vi "Dictionary Set Modified Data__ogtk.vi"(8 "error in (no error)":errorcluster, 10 "Data in":T2, 11 "Object RefNum":T1) -> (0 "error out":errorcluster, 3 "dup Object RefNum":T1)   [LabVIEW 2019]
doc: "Sets the GOOP data structure and releases mutex"
uses:
  Dictionary Object Data Core Task Enum__ogtk.ctl
  Dictionary Data__ogtk.ctl
  Dictionary Object RefNum - Enum__ogtk.ctl
  Dictionary Object RefNum__ogtk.ctl
panel:
  # "OpenGOOP Set Modified Data.vi\n\nSets the GOOP data structure and releases mutex\n\nPlease visit http://www.OpenG.org to learn about the\nOpen Source LabVIEW software movement.\n\nNOTICE -- YOU MUST LEAVE THIS NOTICE IN PLACE.  PER THE TERMS OF THE LICENSE BELOW, YOU MAY SUBLICENSE THIS SOFTWARE \nIN ANY WAY THAT DOES NOT CONFLICT WITH THIS LICENSE.\n\n### BSD License (http://www.opensource.org/licenses/bsd-license.php) Begin ###\n \nCopyright (c) 2003, Jim Kring <jim@jimkring.com>\n\nAll rights reserved.\n\nRedistribution and use in source and binary forms, with or without modification, are permitted provided that the following conditions are met:\n\n    * Redistributions of source code must retain the above copyright notice, this list of conditions and the following disclaimer.\n    * Redistributions in binary form must reproduce the above copyright notice, this list of conditions and the following disclaimer in the \n       documentation and/or other materials provided with the distribution.\n    * Neither the name of SciWare, James Kring, Inc., nor the names of its contributors may be used to endorse or promote products derived \n       from this software without specific prior written permission.\n\nTHIS SOFTWARE IS PROVIDED BY THE COPYRIGHT HOLDERS AND CONTRIBUTORS \"AS IS\" AND ANY EXPRESS OR IMPLIED WARRANTIES, \nINCLUDING, BUT NOT LIMITED TO, THE IMPLIED WARRANTIES OF MERCHANTABILITY AND FITNESS FOR A PARTICULAR PURPOSE ARE \nDISCLAIMED. IN NO EVENT SHALL THE COPYRIGHT OWNER OR CONTRIBUTORS BE LIABLE FOR ANY DIRECT, INDIRECT, INCIDENTAL,\n SPECIAL, EXEMPLARY, OR CONSEQUENTIAL DAMAGES (INCLUDING, BUT NOT LIMITED TO, PROCUREMENT OF SUBSTITUTE GOODS OR \nSERVICES; LOSS OF USE, DATA, OR PROFITS; OR BUSINESS INTERRUPTION) HOWEVER CAUSED AND ON ANY THEORY OF LIABILITY, \nWHETHER IN CONTRACT, STRICT LIABILITY, OR TORT (INCLUDING NEGLIGENCE OR OTHERWISE) ARISING IN ANY WAY OUT OF THE USE \nOF THIS SOFTWARE, EVEN IF ADVISED OF THE POSSIBILITY OF SUCH DAMAGE.\n\n### BSD License End ###"
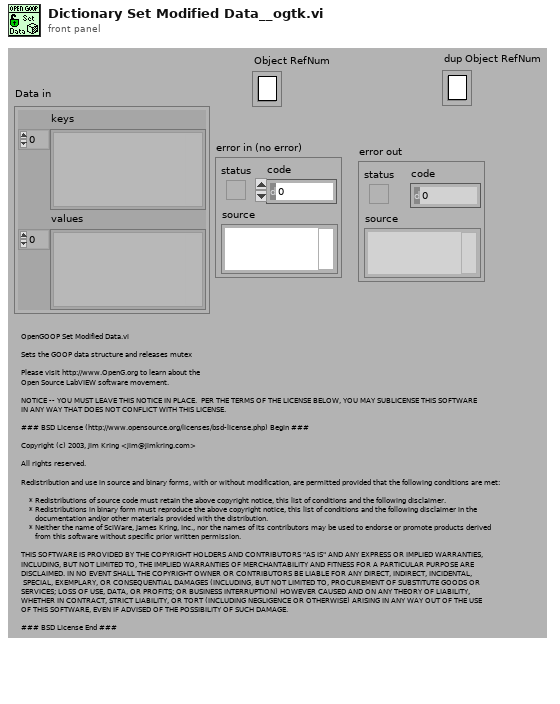
[diagram p1: front panel]
types:
  T1 = typedef "Dictionary Object RefNum__ogtk.ctl" = refnum<k1>
  T2 = typedef "Dictionary Data__ogtk.ctl" = cluster{"keys":variant[], "values":variant[]}
  T3 = typedef "Dictionary Object Data Core Task Enum__ogtk.ctl" = enum16{"read", "write", "init"}
  T4 = typedef "Semaphore RefNum" = refnum<k1>
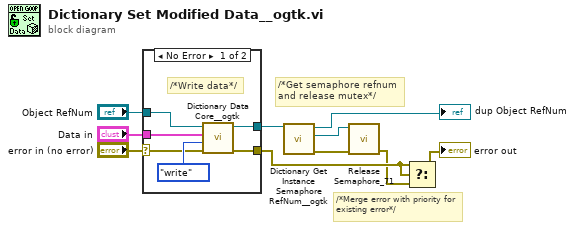
[diagram p0: block diagram]
diagram:
  # "/*Merge error with priority for existing error*/"
  # "/*Get semaphore refnum and release mutex*/"
  n1 = case shown="No Error" "error in (no error)" {
    selector: "error in (no error)" -> [w15 w18]
    tunnel: [w12 w18] -> w4
    tunnel: "Data in" -> [w14 _]
    tunnel: "Object RefNum" -> [w13 w17]
    tunnel: [w11 w17] -> w5
    frame No Error {
      # "/*Write data*/"
      n2 = call "Dictionary Data Core__ogtk.vi"("error in (no error)"=w15, "task (read)"=Dictionary_Object_Data_Core_Task_Enum__ogtk."write", "Data in"=w14, "Object RefNum"=w13) -> ("error out"=w12:errorcluster, "dup Object RefNum"=w11:T1)  [unwired: 5 in, 1 out]
    }
    frame Error {
    }
  }
  n3 = call "Dictionary Get Instance Semaphore RefNum__ogtk.vi"("Object RefNum"=w5) -> ("error in (no error)"=w7:errorcluster, "semaphore"=w6:T4, "dup Object RefNum"=→"dup Object RefNum":T1)  [unwired: 8 in]
  n4 = call <vilib>:"Release Semaphore_71.vi"("error in (no error)"=w7, "semaphore"=w6) -> ("error out"=w3:errorcluster)  [unwired: 4 in, 1 out]
  n5 = Select(t=w4, s=w4, f=w3) -> (s? t:f=→"error out":errorcluster)
